vi "Init Section Views.vi"(4 "Z Scale.Marker Values[]":cluster{"Numeric":dbl, "Numeric":u32}[](array[cluster]), 7 "Graphs":T1, 8 "error in":errorcluster, 9 "Image Size":cluster{"Rows":u32, "Cols":u32}, 11 "Detail Graph.lvclass":refnum<class "Graph with Section Views.lvclass">) -> (0 "error out":errorcluster, 3 "Detail Graph out.lvclass":refnum<class "Graph with Section Views.lvclass">)   [LabVIEW 2023, in "Graph with Section Views.lvclass"]
uses:
  Graph with Section Views.lvclass
  Graph with Section Views.lvclass/Graph with Section Views.ctl
  Base Graph/Base Graph.lvclass
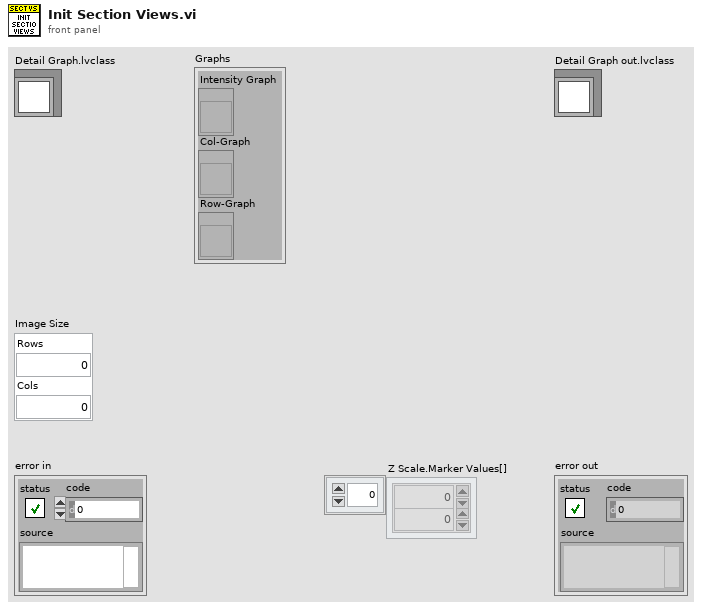
[diagram p1: front panel]
types:
  T1 = cluster{"Intensity Graph":refnum<vi>, "Col-Graph":refnum<vi>, "Row-Graph":refnum<vi>}
  T2 = typedef "LVRectTypeDef.ctl" = cluster{"Left":i16, "Top":i16, "Right":i16, "Bottom":i16}
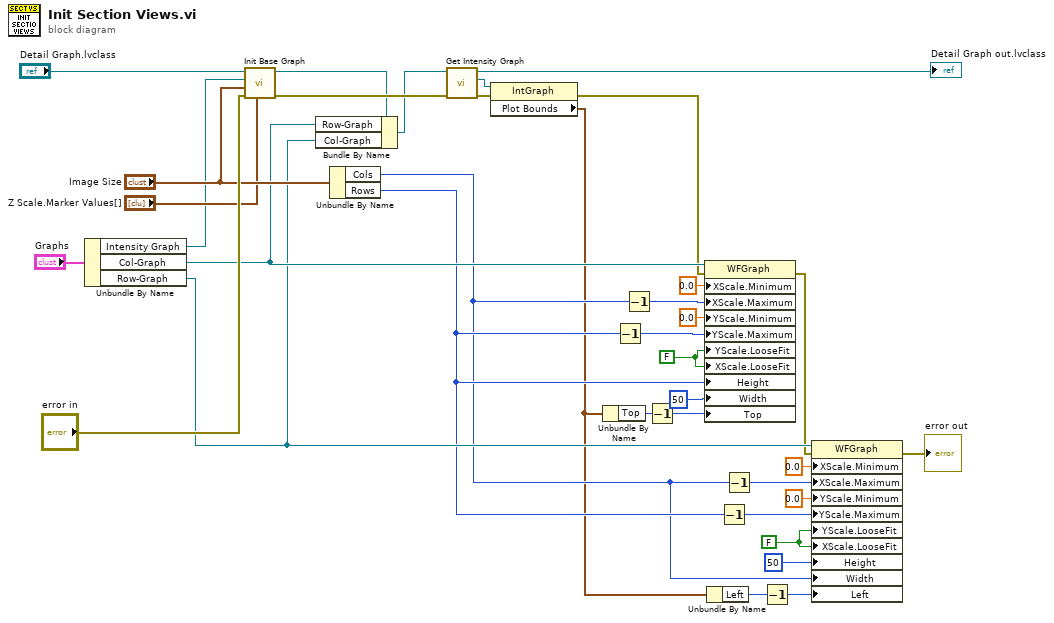
[diagram p0: block diagram]
diagram:
  w20 = FALSE ("Y Scale.Loose Fit")
  w21 = FALSE ("Y Scale.Loose Fit")
  n1 = Unbundle By Name("Graphs") -> ("Intensity Graph"=w31:refnum<vi>, "Col-Graph"=w30:refnum<vi>, "Row-Graph"=w29:refnum<vi>)
  n2 = call "Init Base Graph.vi"("Z Scale.Marker Values[]"="Z Scale.Marker Values[]", "error in"="error in", "Size"="Image Size", "Intensity Graph"=w31, "Base Graph in"="Detail Graph.lvclass") -> ("error out"=w11:errorcluster, "Base Graph out"=w7:refnum<class "Graph with Section Views.lvclass">)  [unwired: 5 in]
  n3 = Bundle By Name(cluster=w7, "Row-Graph"=w30, "Col-Graph"=w29) -> (w6:refnum<class "Graph with Section Views.lvclass">)
  n4 = Unbundle By Name("Image Size") -> ("Cols"=w16:u32, "Rows"=w19:u32)
  n5 = call "Get Intensity Graph.vi"("Base Graph in"=w6) -> ("Intensity Graph"=w9:refnum<vi>, "Base Graph out"=→"Detail Graph out.lvclass":refnum<class "Graph with Section Views.lvclass">)  [unwired: 9 in]
  n6 = property class="IntGraph"(reference=w9, error in=w11) -> (error out=w10:errorcluster, "Plot Bounds"=w4:T2)  [unwired: 1 out]
  n7 = Unbundle By Name(w4) -> ("Top"=w3:i16)
  n8 = Decrement(x=w19) -> (x-1=w15:u32)
  n9 = Decrement(x=w16) -> (x-1=w14:u32)
  n10 = Decrement(x=w3) -> (x-1=w1:i16)
  n11 = property class="WFGraph"(reference=w30, error in=w10, "XScale.Minimum"=0.0 ("X Scale.Range:Minimum"), "XScale.Maximum"=w14, "YScale.Minimum"=0.0 ("Y Scale.Range:Minimum"), "YScale.Maximum"=w15, "YScale.LooseFit"=w21, "XScale.LooseFit"=w21, "Height"=w19, "Width"=u32 50 ("Plot Area:Size:Width"), "Top"=w1) -> (error out=w22:errorcluster)  [unwired: 1 out]
  n12 = Unbundle By Name(w4) -> ("Left"=w5:i16)
  n13 = Decrement(x=w19) -> (x-1=w12:u32)
  n14 = Decrement(x=w16) -> (x-1=w13:u32)
  n15 = Decrement(x=w5) -> (x-1=w2:i16)
  n16 = property class="WFGraph"(reference=w29, error in=w22, "XScale.Minimum"=0.0 ("X Scale.Range:Minimum"), "XScale.Maximum"=w13, "YScale.Minimum"=0.0 ("Y Scale.Range:Minimum"), "YScale.Maximum"=w12, "YScale.LooseFit"=w20, "XScale.LooseFit"=w20, "Height"=u32 50 ("Plot Area:Size:Height"), "Width"=w16, "Left"=w2) -> (error out=→"error out":errorcluster)  [unwired: 1 out]
